vi "set tuner gain mode.vi"(8 "error in (no error)":errorcluster, 10 "manual":i32, 11 "DevRefnum":u64) -> (0 "error out":errorcluster, 3 "DevRefnum":u64)   [LabVIEW 2013, in "rtlsdr.lvlib"]
doc: "RTLSDR_API int rtlsdr_set_tuner_gain_mode(rtlsdr_dev_t *dev, int manual);"
uses:
  rtlsdr.lvlib
  rtlsdr.dll
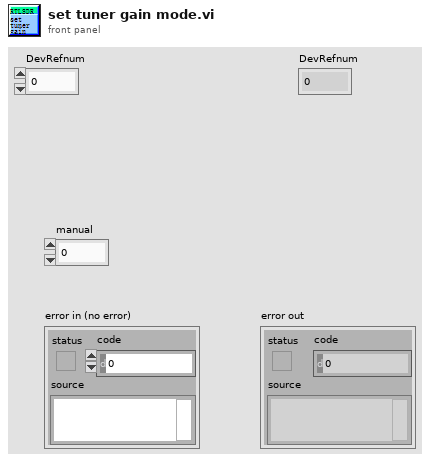
[diagram p1: front panel]
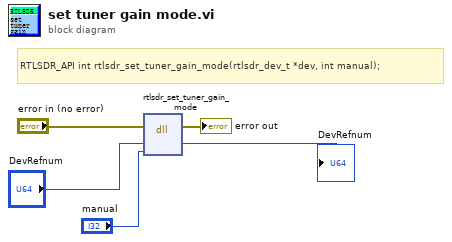
[diagram p0: block diagram]
diagram:
  # "RTLSDR_API int rtlsdr_set_tuner_gain_mode(rtlsdr_dev_t *dev, int manual);"
  n1 = dll-call lib="D:/SDRDriver/Lab1/rtlsdr.*" fn="rtlsdr_set_tuner_gain_mode"(error in="error in (no error)", "DevRefnum"="DevRefnum", "manual"="manual") -> (error out=→"error out":errorcluster, "DevRefnum"=→"DevRefnum":u64)  [unwired: 4 in, 1 out]
